vi "DB - [Schema].[Table].vi"(4 "[PlantId]":string="4070", 5 "Admin User Enum":T1, 6 "DB.Schema.Table 3":string="SRTRS.Config.UserStationAccess", 7 "DB Connection":T3={"Open"=TRUE, "Close"=TRUE}, 8 "error in (no error)":errorcluster, 9 "DB.Schema.Table 2":string="SRTRS.Config.TabUserAccess", 10 "DB.Schema.Table":string="SRTRS.Config.TableGroupType", 11 "connection reference":T2) -> (0 "SUMMARY":errorcluster, 2 "data":string[][](array[string]), 3 "connection reference":T2)   [LabVIEW 2013]
uses:
  <vilib>/addons/database/NI_Database_API.lvlib
  Controls/Global SRTRS.vi
  <vilib>/addons/database/Connection.llb/Conn Execute.vi
  <vilib>/addons/database/Recordset.llb/Rec Destroy - Connection.vi
  <vilib>/addons/database/Recordset.llb/Rec Fetch Recordset Data (R).vi
  <vilib>/addons/database/_DB Variant To Data/Database Variant To Data.xnode
  <vilib>/addons/database/Connection.llb/DB Tools Open Connec (Path).vi
  <vilib>/addons/database/Connection.llb/Conn ObjectReference.ctl
  Controls/DB - OpenClose.ctl
  Controls/DB - Admin User Enum.ctl
panel:
  out "SQL Statement":string
  out "Connection Information":T4={"Connection "="SQL Server 32bit HPEnvy", "Username"="admin", "Password"="admin123"}
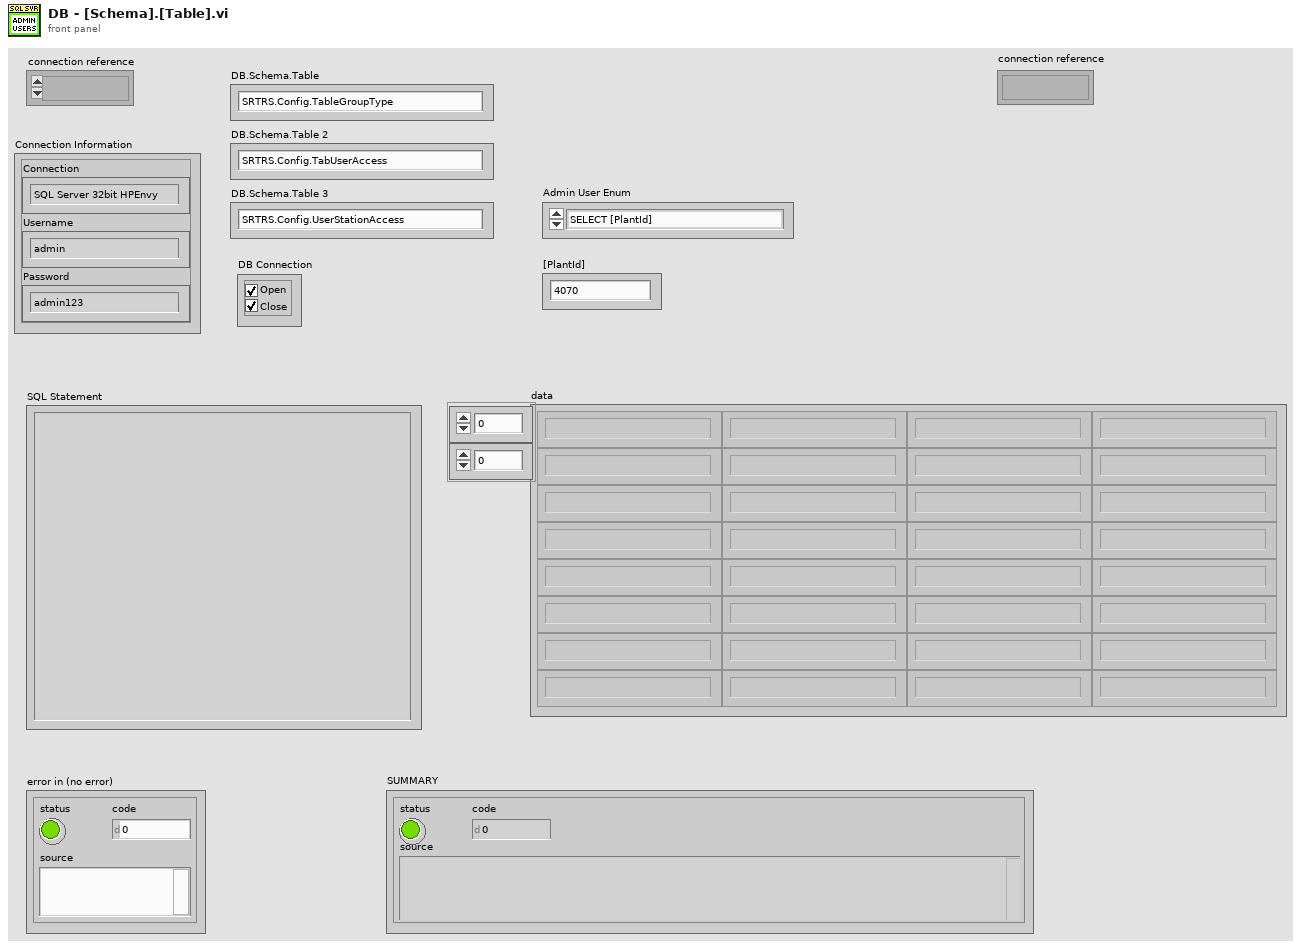
[diagram p1: front panel]
types:
  T1 = typedef "DB - Admin User Enum.ctl" = enum16{"SELECT [PlantId]", "UPDATE [PlantId],[UserId]", "INSERT [PlantId],[UserId]"}
  T2 = typedef "NI_Database_API.lvlib/Conn ObjectReference.ctl" = refnum<k1>
  T3 = typedef "DB - OpenClose.ctl" = cluster{"Open":bool, "Close":bool}
  T4 = cluster{"Connection ":string, "Username":string, "Password":string}
  T5 = typedef "Enum - InteractiveMode-SubVIMode.ctl" = enum16{"Interactive", "subVI Mode"}
  T6 = typedef "DB - DB.Schema.Table.ctl" = cluster{"DB":string, "Schema":string, "Table":string}
  T7 = typedef "NI_Database_API.lvlib/Rec ObjectReference.ctl" = refnum<k1>
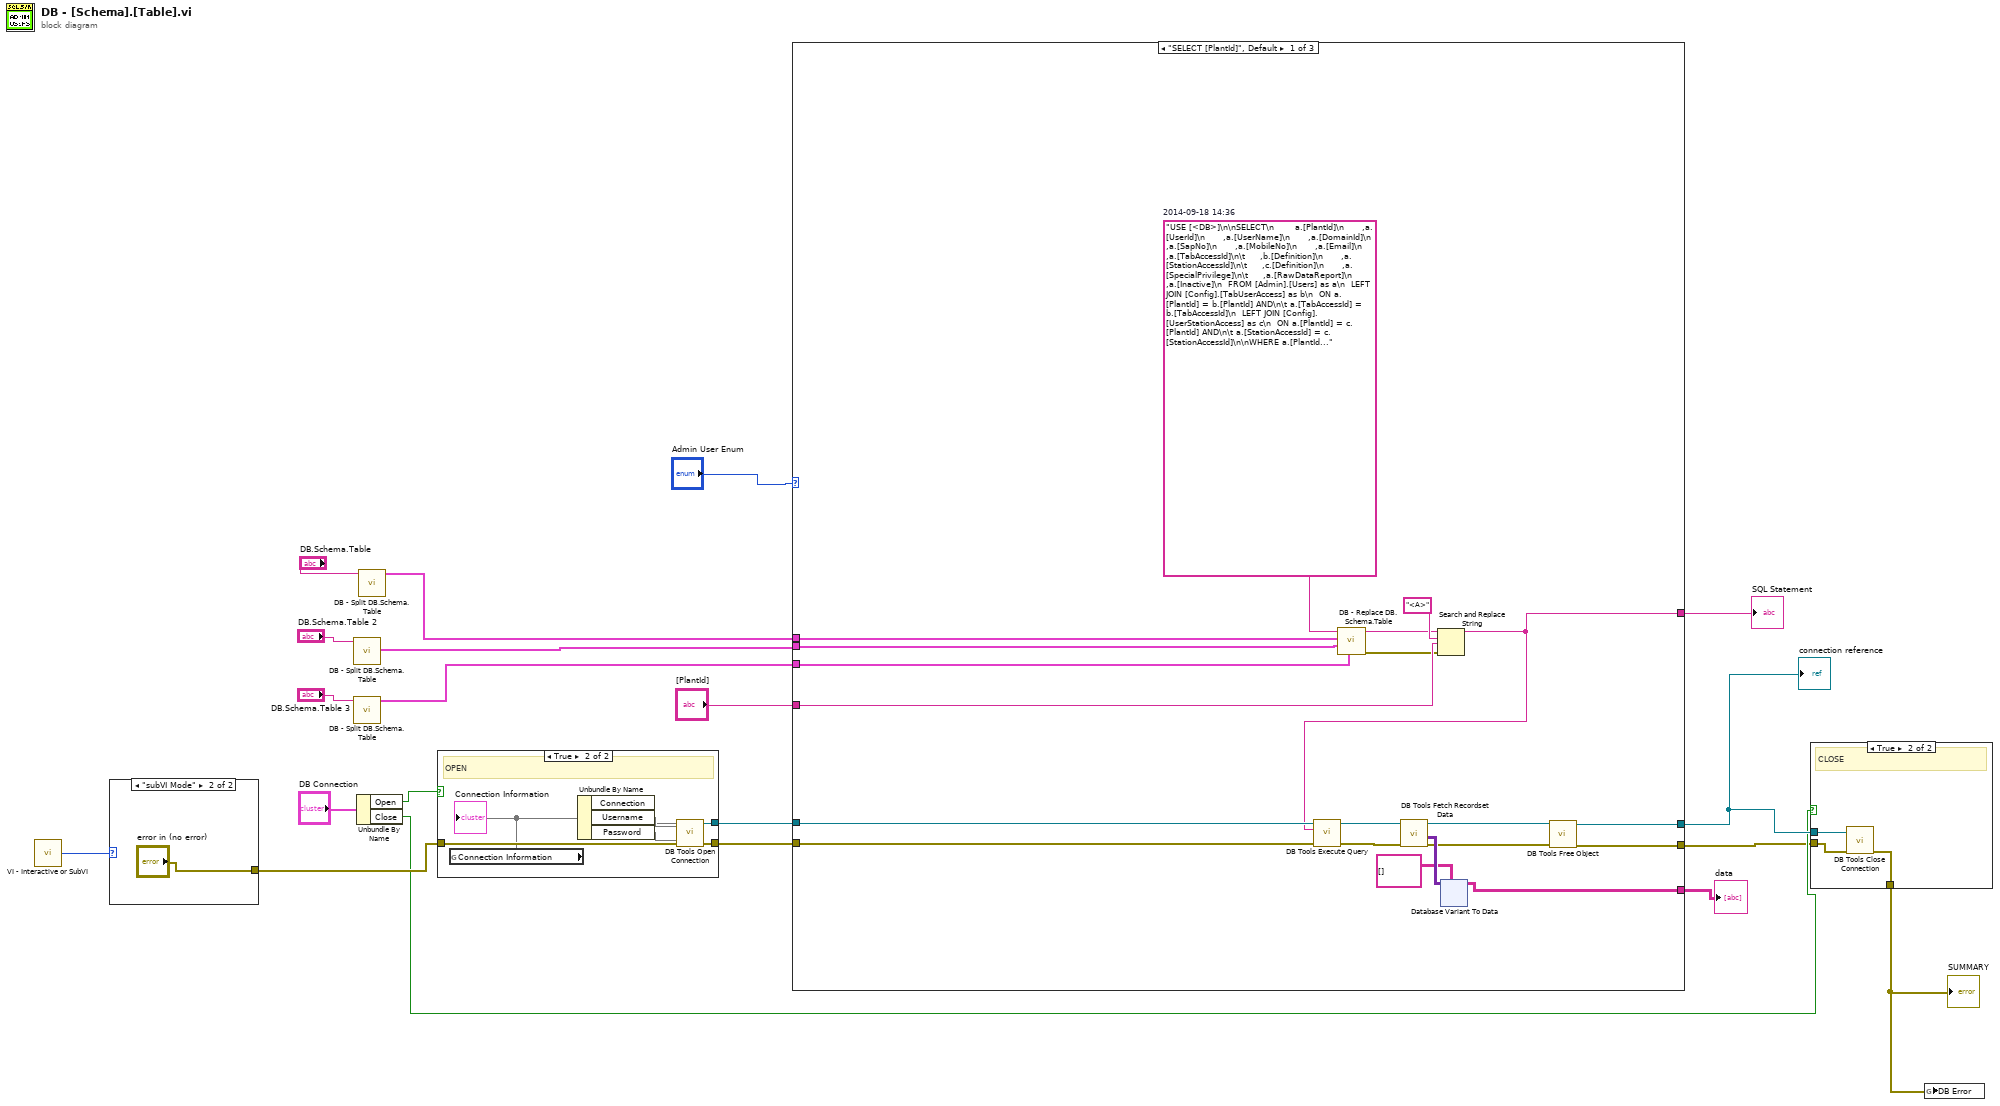
[diagram p0: block diagram]
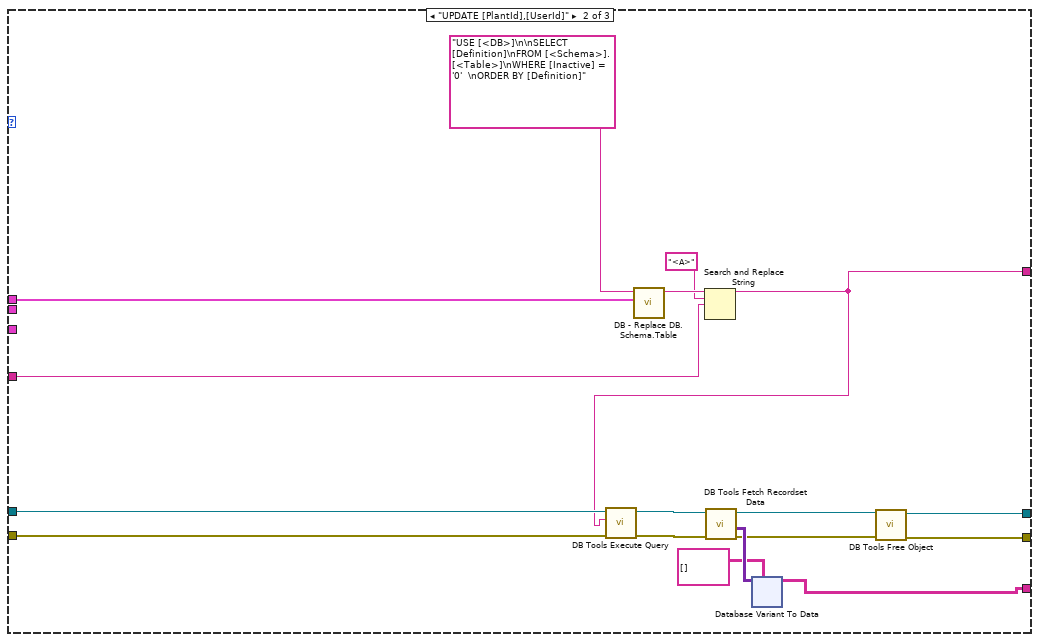
[diagram p2: hidden frame]
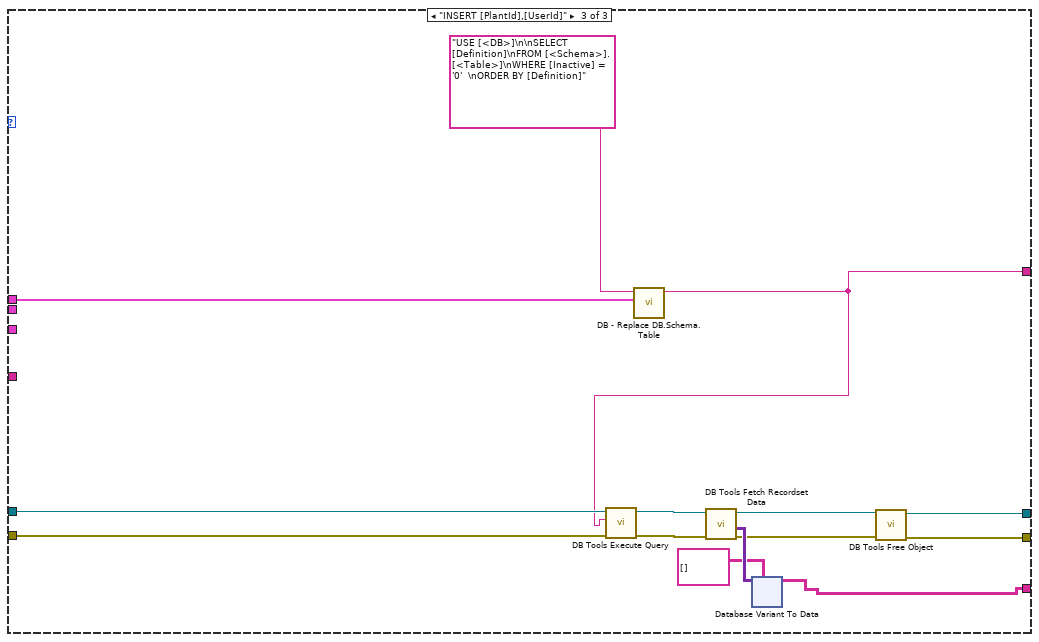
[diagram p3: hidden frame]
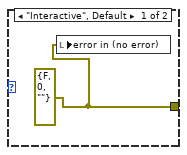
[diagram p5: hidden frame]
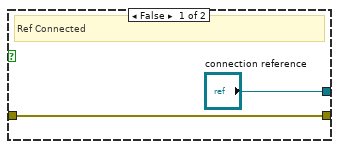
[diagram p6: hidden frame]
diagram:
  n1 = call "VI - Interactive or SubVI.vi"() -> ("Mode"=w18:T5)  [unwired: 5 in]
  n2 = case shown="\"subVI Mode\"" w18 {
    tunnel: [w21 "error in (no error)"] -> w17
    frame "Interactive", Default {
      w21 = errorcluster {"status"=FALSE, "code"=0, "source"=""} ("error in (no error)")
      n3 = local write "error in (no error)"(w21) -> ()
    }
    frame "subVI Mode" {
    }
  }
  n4 = call "DB - Split DB.Schema.Table.vi"("DB.Schema.Table"="DB.Schema.Table 2") -> ("DB.Schema.Table"=w5:T6)  [unwired: 10 in]
  n5 = call "DB - Split DB.Schema.Table.vi"("DB.Schema.Table"="DB.Schema.Table 3") -> ("DB.Schema.Table"=w4:T6)  [unwired: 10 in]
  n6 = Unbundle By Name("DB Connection") -> ("Open"=w19:bool, "Close"=w13:bool)
  n7 = call "DB - Split DB.Schema.Table.vi"("DB.Schema.Table"="DB.Schema.Table") -> ("DB.Schema.Table"=w9:T6)  [unwired: 10 in]
  n8 = case shown="True" w19 {
    tunnel: ["connection reference" w28] -> w16
    tunnel: w17 -> [w23 w27]
    tunnel: [w23 w26] -> w15
    frame False {
      # "Ref Connected"
    }
    frame True {
      # "OPEN"
      n9 = global read "Global SRTRS.vi" "Connection Information"() -> (w25)
      "Connection Information" <- w25
      n10 = Unbundle By Name(w25) -> ("Connection"=w30, "Username"=w31, "Password"=w29)
      n11 = call-poly <vilib>:"DB Tools Open Connection.vi"("password"=w29, "userID"=w31, "error in (no error)"=w27, "connection information"=w30) -> ("error out"=w26:errorcluster, "connection reference"=w28:T2)  [unwired: 4 in]
    }
  }
  n12 = case shown="\"SELECT [PlantId]\", Default" "Admin User Enum" {
    tunnel: w16 -> [w45 w106 w164]
    tunnel: w15 -> [w44 w105 w163]
    tunnel: [w43 w104 w162] -> w14
    tunnel: [w42 w103 w161] -> w12
    tunnel: w9 -> [w41 w102 w160]
    tunnel: [w34 w98 w159] -> w8
    tunnel: w5 -> [w39 _ _]
    tunnel: w4 -> [w38 _ _]
    tunnel: [w37 w100 w157] -> w3
    tunnel: "[PlantId]" -> [w33 w96 _]
    frame "SELECT [PlantId]", Default {
      w40 = "USE [<DB>]\n\nSELECT\n       a.[PlantId]\n      ,a.[UserId]\n      ,a.[UserName]\n      ,a.[DomainId]\n      ,a.[SapNo]\n      ,a.[MobileNo]\n      ,a.[Email]\n      ,a.[TabAccessId]\n\t     ,b.[Definition]\n      ,a.[StationAccessId]\n\t     ,c.[Definition]\n      ,a.[SpecialPrivilege]\n\t     ,a.[RawDataReport]\n      ,a.[Inactive]\n  FROM [Admin].[Users] as a\n  LEFT JOIN [Config].[TabUserAccess] as b\n  ON a.[PlantId] = b.[PlantId] AND\n\t a.[TabAccessId] = b.[TabAccessId]\n  LEFT JOIN [Config].[UserStationAccess] as c\n  ON a.[PlantId] = c.[PlantId] AND\n\t a.[StationAccessId] = c.[StationAccessId]\n\nWHERE a.[PlantId] = '<A>'\n"  # 2014-09-18 14:36
      n13 = call "DB - Replace DB.Schema.Table.vi"("DB.Schema.Table 3"=w38, "DB.Schema.Table 2"=w39, "DB.Schema.Table"=w41, "string in"=w40) -> ("error out"=w32:errorcluster, "string out"=w35:string)  [unwired: 6 in]
      n14 = Search and Replace String(input string=w35, search string="<A>", replace string=w33, error in=w32) -> (result string=w34:string)  [unwired: 4 in, 3 out]
      n15 = call-poly <vilib>:"DB Tools Execute Query.vi"("error in (no error)"=w44, "SQL query"=w34, "connection reference"=w45) -> ("error out"=w51:errorcluster, "recordset reference"=w50:T7)  [unwired: 5 in]
      n16 = call-poly <vilib>:"DB Tools Fetch Recordset Data.vi"("error in (no error)"=w51, "recordset reference"=w50) -> ("error out"=w46:errorcluster, "recordset data"=w49:variant[][], "recordset reference out"=w47:T7)  [unwired: 3 in]
      n17 = xnode "Database Variant To Data"("database variant"=w49, "type"=string[][] []) -> ("data"=w37:string[][])  [unwired: 1 in, 1 out]
      n18 = call-poly <vilib>:"DB Tools Free Object.vi"("error in (no error)"=w46, "recordset reference"=w47) -> ("error out"=w42:errorcluster, "connection reference"=w43:T2)  [unwired: 8 in]
    }
    frame "UPDATE [PlantId],[UserId]" {
      n19 = call "DB - Replace DB.Schema.Table.vi"("DB.Schema.Table"=w102, "string in"="USE [<DB>]\n\nSELECT [Definition]\nFROM [<Schema>].[<Table>]\nWHERE [Inactive] = '0'  \nORDER BY [Definition]" ("SQL query")) -> ("string out"=w99:string)  [unwired: 8 in, 1 out]
      n20 = Search and Replace String(input string=w99, search string="<A>", replace string=w96) -> (result string=w98:string)  [unwired: 5 in, 3 out]
      n21 = call-poly <vilib>:"DB Tools Execute Query.vi"("error in (no error)"=w105, "SQL query"=w98, "connection reference"=w106) -> ("error out"=w112:errorcluster, "recordset reference"=w111:T7)  [unwired: 5 in]
      n22 = call-poly <vilib>:"DB Tools Fetch Recordset Data.vi"("error in (no error)"=w112, "recordset reference"=w111) -> ("error out"=w107:errorcluster, "recordset data"=w110:variant[][], "recordset reference out"=w108:T7)  [unwired: 3 in]
      n23 = xnode "Database Variant To Data"("database variant"=w110, "type"=string[][] []) -> ("data"=w100:string[][])  [unwired: 1 in, 1 out]
      n24 = call-poly <vilib>:"DB Tools Free Object.vi"("error in (no error)"=w107, "recordset reference"=w108) -> ("error out"=w103:errorcluster, "connection reference"=w104:T2)  [unwired: 8 in]
    }
    frame "INSERT [PlantId],[UserId]" {
      n25 = call "DB - Replace DB.Schema.Table.vi"("DB.Schema.Table"=w160, "string in"="USE [<DB>]\n\nSELECT [Definition]\nFROM [<Schema>].[<Table>]\nWHERE [Inactive] = '0'  \nORDER BY [Definition]" ("SQL query")) -> ("string out"=w159:string)  [unwired: 8 in, 1 out]
      n26 = call-poly <vilib>:"DB Tools Execute Query.vi"("error in (no error)"=w163, "SQL query"=w159, "connection reference"=w164) -> ("error out"=w170:errorcluster, "recordset reference"=w169:T7)  [unwired: 5 in]
      n27 = call-poly <vilib>:"DB Tools Fetch Recordset Data.vi"("error in (no error)"=w170, "recordset reference"=w169) -> ("error out"=w165:errorcluster, "recordset data"=w168:variant[][], "recordset reference out"=w166:T7)  [unwired: 3 in]
      n28 = xnode "Database Variant To Data"("database variant"=w168, "type"=string[][] []) -> ("data"=w157:string[][])  [unwired: 1 in, 1 out]
      n29 = call-poly <vilib>:"DB Tools Free Object.vi"("error in (no error)"=w165, "recordset reference"=w166) -> ("error out"=w161:errorcluster, "connection reference"=w162:T2)  [unwired: 8 in]
    }
  }
  "connection reference" <- w14
  "SQL Statement" <- w8
  "data" <- w3
  n30 = case shown="True" w13 {
    tunnel: [w215 w217] -> w1
    tunnel: w14 -> [_ w218]
    tunnel: w12 -> [w215 w216]
    frame False {
      # "Ref Connected"
    }
    frame True {
      # "CLOSE"
      n31 = call <vilib>:"DB Tools Close Connection.vi"("error in (no error)"=w216, "connection reference"=w218) -> ("error out"=w217:errorcluster)  [unwired: 5 in]
    }
  }
  "SUMMARY" <- w1
  n32 = global write "Global SRTRS.vi" "DB Error"(w1) -> ()
